vi "Configure Frequency Shift.vi"(0 "niUsrpRio session":T1 {"Daughterboard Clock Rate" format="%#.3pHz"; "FPGA Data Clock Rate" format="%#.3pHz"; "Data Clock Rate" format="%#.3pHz"; "Characterization Data"."Frequencies [Hz]" format="%#_6p"; "EEPROM Characterization Header"."Pointer to Device Data Header" format="%x"; "EEPROM Characterization Header"."Checksum" format="%x"; "Device Data Header"."Pointer to Characterization Data" format="%x"; "Device Data Header"."Checksum" format="%x"; "EEPROM Header"."Pointer to User Header" format="%x"; "EEPROM Header"."Pointer to Factory Header" format="%x"; "EEPROM Header"."Product Code" format="%x"; "EEPROM Header"."Checksum" format="%x"}, 1 "scope":string(combo)="rx/RF 0", 5 "frequency shift":dbl format="%#.3pHz", 7 "if frequency shift":dbl format="%#.3pHz", 11 "error in":errorcluster) -> (4 "niUsrpRio Session (out)":T1={"FPGA Interface"=refnum, "RIO Interface Number"=0, "Data Clock Rate"=0, "FPGA Data Clock Rate"=0, "Global Settings Register Bus"=refnum, "Radio 0 Settings Register Bus"=refnum, "Radio 1 Settings Register Bus"=refnum, "Radio Settings Bus Semaphore"=refnum, "DB Queues"=[], "Characterization Data Valid?"=FALSE, "EEPROM Header"={"Checksum"=0, "Product Code"=0, "Hardware Current Version"=0, "Hardware Oldest Compatible Version"=0, "EEPROM Map Current Version"=0, "EEPROM Map Oldest Compatible Version"=0, "User Password"="", "Pointer to Factory Header"=0, "Pointer to User Header"=0, "Recommended Interval"=0, "Number of Reserved Bytes"=9, "Number of Daughterboards"=0, "Daughterboard IDs"=[], "Daughterboard Serial Numbers"=[]}, "Device Data Header"={"Checksum"=0, "Number of Channels"=0, "Number of Gain Settings"=[], "Pointer to Characterization Data"=[], "Number of Reserved Bytes"=27, "Number of Frequencies"=[]}, "EEPROM Characterization Header"={"Checksum"=0, "Date"=timestamp(0 s since 1904-01-01), "Temperature"=0.0, "Misc. Info"="", "Pointer to Device Data Header"=0, "Number of Reserved Bytes"=28}, "Characterization Data"=[], "FPGA Current Version"=0, "FPGA Oldest Compatible Version"=0, "Fixed Logic Current Version"=0, "Fixed Logic Oldest Compatible Version"=0, "FPGA Radio Settings Bus Current Version"=0, "FPGA Radio Settings Bus Oldest Compatible Version"=0, "FPGA Board Config Current Version"=0, "FPGA Board Config Oldest Compatible Version"=0, "Daughterboard Clock Rate"=0, "daughterboard configuration session handles"=[]} {"Daughterboard Clock Rate" format="%#.3pHz"; "FPGA Data Clock Rate" format="%#.3pHz"; "Data Clock Rate" format="%#.3pHz"; "Characterization Data"."Frequencies [Hz]" format="%#_6p"; "EEPROM Characterization Header"."Pointer to Device Data Header" format="%x"; "EEPROM Characterization Header"."Checksum" format="%x"; "Device Data Header"."Pointer to Characterization Data" format="%x"; "Device Data Header"."Checksum" format="%x"; "EEPROM Header"."Pointer to User Header" format="%x"; "EEPROM Header"."Pointer to Factory Header" format="%x"; "EEPROM Header"."Product Code" format="%x"; "EEPROM Header"."Checksum" format="%x"}, 6 "coerced frequency shift":dbl format="%#.3pHz", 8 "if coerced frequency shift":dbl format="%#.3pHz", 15 "error out":errorcluster)   [LabVIEW 2018]
doc: "Configures the digital frequency shift amount.\n\n<B>Input Parameters</B>\n\n<B>niUsrpRio Session</B> is the object created by the Open VI and used as the session handle for the USRP RIO design library.\n\n<B>clock rate</B> is the frequency, in hertz, at which the DSP blocks run.\n\n<B>frequency shift</B> is the amount, in hertz, by which to shift the frequency.\n\n<B>error in</B> describes error conditions that occur before this node runs. This input provides standard 'error in' functionality.\n\n<B>Output Parameters</B>\n\n<B>error out</B> contains error information. This output provides standard 'error out' functionality."
uses:
  <instrlib>/niUsrpRio/Config/v1/Host/Public/niUsrpRio Session.ctl
  <instrlib>/_niInstr/Register Bus/v0/Host/Public/Register Bus Session.ctl
  <instrlib>/_niInstr/Register Bus/v0/Host/Private/Session Data.ctl
  <instrlib>/niUsrpRio/Config/v1/Host/Private/DB Queue Reference.ctl
  <instrlib>/niUsrpRio/Config/v1/Host/Private/Daughterboard Data.ctl
  <instrlib>/niUsrpRio/Config/v1/Host/Private/ATR state data.ctl
  <instrlib>/niUsrpRio/Config/v1/Host/Private/Antenna Configuration.ctl
  <instrlib>/niUsrpRio/Config/v1/Host/Private/CPLD Power Mode.ctl
  <instrlib>/niUsrpRio/Config/v1/Host/Public/EEPROM Header.ctl
  <instrlib>/niUsrpRio/Config/v1/Host/Public/EEPROM Device Data Header.ctl
  <instrlib>/niUsrpRio/Config/v1/Host/Public/EEPROM Characterization Header.ctl
  <instrlib>/niUsrpRio/Config/v1/Host/Public/Characterization Data.ctl
  <instrlib>/niUsrpRio/Config/v1/Host/Public/IQ Imbalance.ctl
  FPGA/SubVIs/DDC Parameters.ctl
  <instrlib>/_niInstr/DSP/v1/Shared/Public/IQ Impairments.ctl
  <vilib>/Utility/error.llb/Error Cluster From Error Code.vi
  <vilib>/rvi/errors/niLvFpgaAdjustHostInterfaceError.vi
  <vilib>/ErrorRing/Error Ring.xnode
  <vilib>/rvi/interface/nirviReadWriteControl/nirviReadWriteControl.xnode
  NiFpgaLv.dll
  <vilib>/rvi/interface/Simulation/niFpgaSimulationCallBeginRW.vi
  <instrlib>/niUsrpRio/Config/v1/Host/niUsrpRio Config v1 Host.lvlib
  <instrlib>/_niInstr/DSP/v1/Shared/niInstr DSP v1 Shared.lvlib
  <instrlib>/_niInstr/Register Bus/v0/Host/niInstr Register Bus v0 Host.lvlib
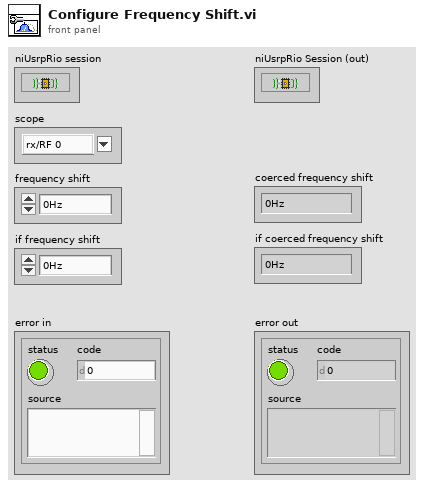
[diagram p1: front panel]
types:
  T1 = typedef "niUsrpRio Config v1 Host.lvlib/niUsrpRio Session.ctl" = cluster{"FPGA Interface":refnum<k20>, "RIO Interface Number":u32, "Data Clock Rate":u32, "FPGA Data Clock Rate":u32, "Global Settings Register Bus":T2, "Radio 0 Settings Register Bus":T2, "Radio 1 Settings Register Bus":T2, "Radio Settings Bus Semaphore":T3, "DB Queues":T4[], "Characterization Data Valid?":bool, "EEPROM Header":T5, "Device Data Header":T6, "EEPROM Characterization Header":T7, "Characterization Data":T8[], "FPGA Current Version":u32, "FPGA Oldest Compatible Version":u32, "Fixed Logic Current Version":u32, "Fixed Logic Oldest Compatible Version":u32, "FPGA Radio Settings Bus Current Version":u32, "FPGA Radio Settings Bus Oldest Compatible Version":u32, "FPGA Board Config Current Version":u32, "FPGA Board Config Oldest Compatible Version":u32, "Daughterboard Clock Rate":u32, "daughterboard configuration session handles":u64[]}
  T2 = typedef "niInstr Register Bus v0 Host.lvlib/Register Bus Session.ctl" = refnum<queue>
  T3 = typedef "Semaphore RefNum" = refnum<k1>
  T4 = typedef "niUsrpRio Config v1 Host.lvlib/DB Queue Reference.ctl" = refnum<queue>
  T5 = typedef "niUsrpRio Config v1 Host.lvlib/EEPROM Header.ctl" = cluster{"Checksum":u32, "Product Code":u16, "Hardware Current Version":u16, "Hardware Oldest Compatible Version":u16, "EEPROM Map Current Version":u16, "EEPROM Map Oldest Compatible Version":u16, "User Password":string, "Pointer to Factory Header":u32, "Pointer to User Header":u32, "Recommended Interval":u16, "Number of Reserved Bytes":i32, "Number of Daughterboards":u8, "Daughterboard IDs":u16[], "Daughterboard Serial Numbers":string[]}
  T6 = typedef "niUsrpRio Config v1 Host.lvlib/EEPROM Device Data Header.ctl" = cluster{"Checksum":u32, "Number of Channels":u8, "Number of Gain Settings":u16[], "Pointer to Characterization Data":u32[], "Number of Reserved Bytes":i32, "Number of Frequencies":u16[]}
  T7 = typedef "niUsrpRio Config v1 Host.lvlib/EEPROM Characterization Header.ctl" = cluster{"Checksum":u32, "Date":timestamp, "Temperature":sgl, "Misc. Info":string, "Pointer to Device Data Header":u32, "Number of Reserved Bytes":i32}
  T8 = typedef "niUsrpRio Config v1 Host.lvlib/Characterization Data.ctl" = cluster{"Gains[dB]":dbl[], "Frequencies [Hz]":dbl[], "IQ Imbalance Table":T9[], "Measured Gains[dB]":dbl[][]}
  T9 = typedef "niUsrpRio Config v1 Host.lvlib/IQ Imbalance.ctl" = cluster{"Gain Imbalance [linear]":dbl, "Phase Imbalance [radians]":dbl, "Offset":cdb}
  T10 = typedef "DDC Parameters.ctl" = cluster{"output sample rate":fxp<+,48,1>, "delay":fxp<+/-,16,0>, "frequency shift":fxp<+/-,48,0>, "impairments":T11, "phase":fxp<+/-,21,0>}
  T11 = typedef "niInstr DSP v1 Shared.lvlib/IQ Impairments.ctl" = cluster{"inline gain I":fxp<+/-,18,1>, "inline gain Q":fxp<+/-,18,1>, "cross gain I":fxp<+/-,18,1>, "cross gain Q":fxp<+/-,18,1>, "pre-gain offset I":fxp<+/-,18,1>, "pre-gain offset Q":fxp<+/-,18,1>, "post-gain offset I":fxp<+/-,18,1>, "post-gain offset Q":fxp<+/-,18,1>}
  T12 = typedef "niUsrpRio Config v1 Host.lvlib/Device Subfunction.ctl" = enum16{"rx", "tx", "all"}
  T13 = typedef "niUsrpRio Config v1 Host.lvlib/RF Channel 2.ctl" = enum16{"0", "1", "2", "3", "All"}
  T14 = typedef "niUsrpRio Config v1 Host.lvlib/DB Types.ctl" = enum16{"sbx", "cbx", "wbx", "unknown", "ubx", "twinrx"}
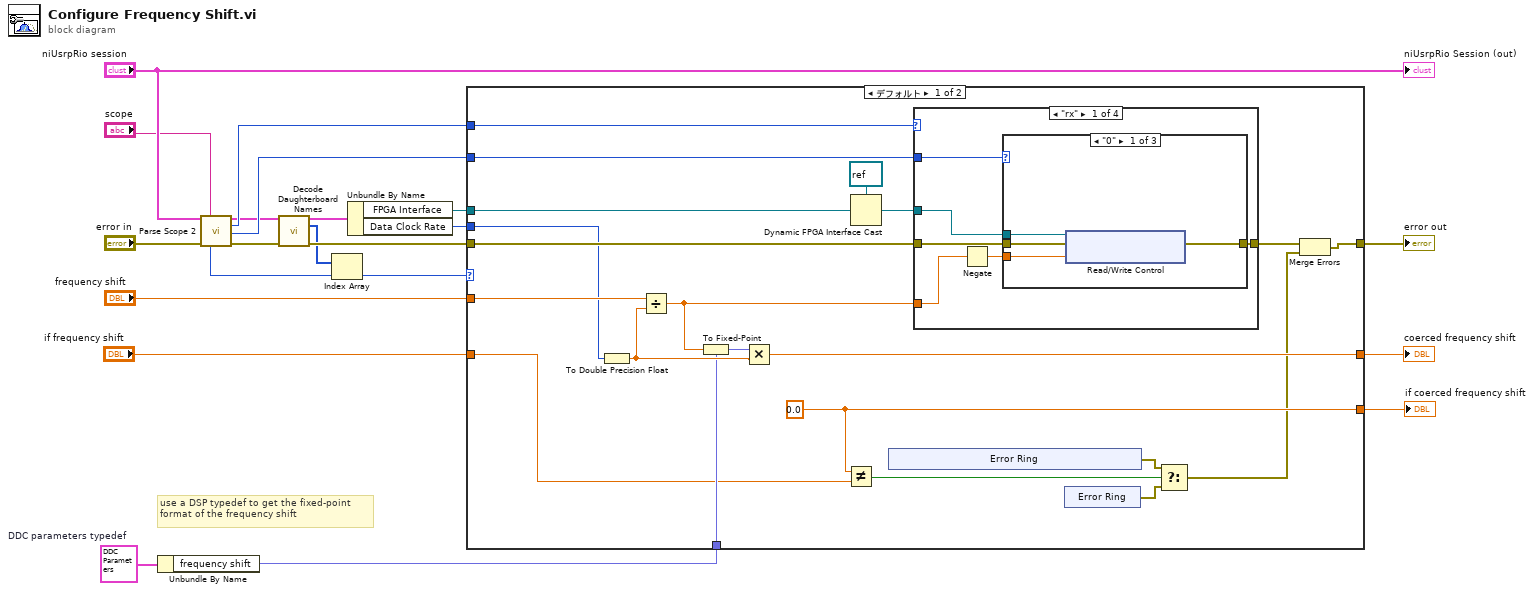
[diagram p0: block diagram]
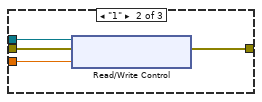
[diagram p2: hidden frame]
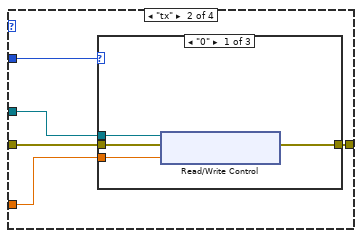
[diagram p4: hidden frame]
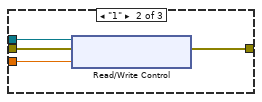
[diagram p5: hidden frame]
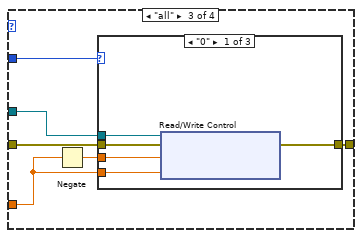
[diagram p7: hidden frame]
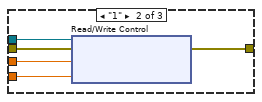
[diagram p8: hidden frame]
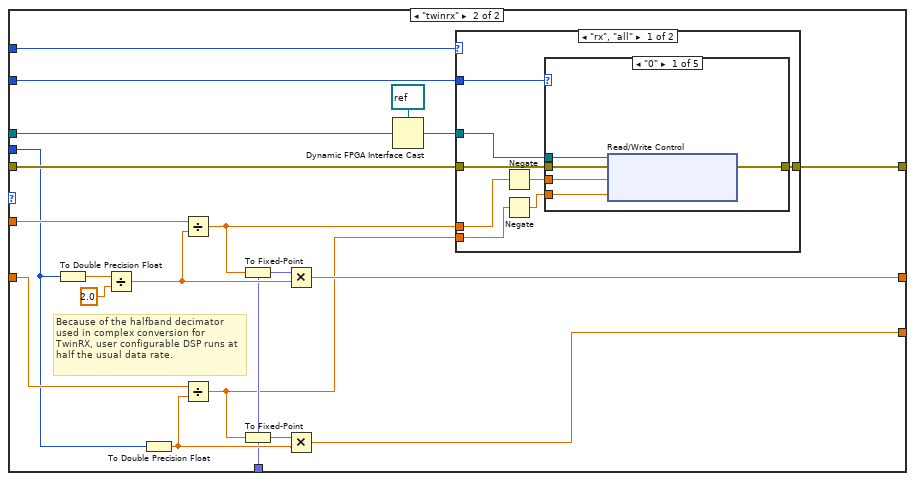
[diagram p11: hidden frame]
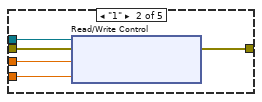
[diagram p12: hidden frame]
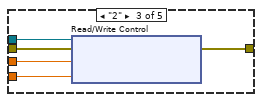
[diagram p13: hidden frame]
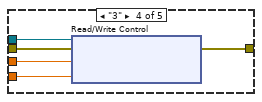
[diagram p14: hidden frame]
diagram:
  w19 = T10 {"output sample rate"=1.0, "delay"=0.0, "frequency shift"=0.0, "impairments"={"inline gain I"=0.9999923706054688, "inline gain Q"=0.9999923706054688, "cross gain I"=0.0, "cross gain Q"=0.0, "pre-gain offset I"=0.0, "pre-gain offset Q"=0.0, "post-gain offset I"=0.0, "post-gain offset Q"=0.0}, "phase"=0.0}  # DDC parameters typedef
  # "use a DSP typedef to get the fixed-point format of the frequency shift"
  n1 = Unbundle By Name(w19) -> ("frequency shift"=w6:fxp<+/-,48,0>)
  n2 = call <instrlib>:"Parse Scope 2.vi"("niUsrpRio Session"="niUsrpRio session", "scope"="scope", "error in"="error in") -> ("niUsrpRio Session (out)"=w12:T1, "Device Subfunction"=w16:T12, "Device Subfunction Channel"=w21:T13, "daughterboard index"=w9:u32, "error out"=w17:errorcluster)  [unwired: 4 in, 4 out]
  n3 = call <instrlib>:"Decode Daughterboard Names.vi"("niUsrpRio Session"=w12, "error in"=w17) -> ("niUsrpRio Session (out)"=w11:T1, "daughterboard names"=w10:T14[], "error out"=w13:errorcluster)  [unwired: 10 in, 1 out]
  n4 = Index Array(array=w10, index=w9) -> (element=w8:T14)
  n5 = Unbundle By Name(w11) -> ("FPGA Interface"=w7:refnum<k20>, "Data Clock Rate"=w2:u32)
  n6 = case shown="デフォルト" w8 {
    tunnel: w21 -> [w42 w116]
    tunnel: [w24 w115] -> w20
    tunnel: w7 -> [w39 w111]
    tunnel: w16 -> [w41 w114]
    tunnel: w13 -> [w40 w113]
    tunnel: w6 -> [w31 w103]
    tunnel: "if frequency shift" -> [w28 w104]
    tunnel: "frequency shift" -> [w34 w102]
    tunnel: [w32 w101] -> w3
    tunnel: w2 -> [w33 w98]
    tunnel: [w29 w96] -> w1
    frame Default {
      w29 = 0.0
      n7 = To Double Precision Float(number=w33) -> (double precision float=w36:dbl)
      n8 = Divide(x=w34, y=w36) -> (x/y=w30:dbl)
      n9 = To Fixed-Point(fixed-point type=w31, number=w30) -> (fixed-point=w35:fxp<+/-,48,0>)
      n10 = Multiply(x=w35, y=w36) -> (x*y=w32:dbl)
      n11 = Not Equal?(x=w29, y=w28) -> (x != y?=w27:bool)
      n12 = Dynamic FPGA Interface Cast(Session In=refnum<k20> refnum ("FPGA VI Reference Out"), Type=w39) -> (Session Out=w38:refnum<k20>)
      n13 = xnode "Error Ring"() -> ("エラー出力"=w26:errorcluster)
      n14 = case shown="\"rx\"" w41 {
        tunnel: w38 -> [w50 w68 w79 _]
        tunnel: [w54 w67 w83 w95] -> w23
        tunnel: w40 -> [w53 w66 w82 w95]
        tunnel: w42 -> [w51 w65 w80 _]
        tunnel: w30 -> [w49 w64 w78 _]
        frame "rx" {
          n15 = Negate(x=w49) -> (-x=w52:dbl)
          n16 = case shown="\"0\"" w51 {
            tunnel: w50 -> [w58 w62 _]
            tunnel: [w57 w61 w63] -> w54
            tunnel: w53 -> [w56 w60 w63]
            tunnel: w52 -> [w55 w59 _]
            frame "0" {
              n17 = xnode "Read/Write Control"("FPGA VIリファレンス入力"=w58, "エラー入力"=w56, "rx 0.frequency shift"=w55) -> ("エラー出力"=w57:errorcluster)  [unwired: 1 out]
            }
            frame "1" {
              n18 = xnode "Read/Write Control"("FPGA VIリファレンス入力"=w62, "エラー入力"=w60, "rx 1.frequency shift"=w59) -> ("エラー出力"=w61:errorcluster)  [unwired: 1 out]
            }
            frame Default {
            }
          }
        }
        frame "tx" {
          n19 = case shown="\"0\"" w65 {
            tunnel: w68 -> [w72 w76 _]
            tunnel: [w71 w75 w77] -> w67
            tunnel: w66 -> [w70 w74 w77]
            tunnel: w64 -> [w69 w73 _]
            frame "0" {
              n20 = xnode "Read/Write Control"("FPGA VIリファレンス入力"=w72, "エラー入力"=w70, "tx 0.frequency shift"=w69) -> ("エラー出力"=w71:errorcluster)  [unwired: 1 out]
            }
            frame "1" {
              n21 = xnode "Read/Write Control"("FPGA VIリファレンス入力"=w76, "エラー入力"=w74, "tx 1.frequency shift"=w73) -> ("エラー出力"=w75:errorcluster)  [unwired: 1 out]
            }
            frame Default {
            }
          }
        }
        frame "all" {
          n22 = Negate(x=w78) -> (-x=w81:dbl)
          n23 = case shown="\"0\"" w80 {
            tunnel: w79 -> [w88 w93 _]
            tunnel: [w87 w92 w94] -> w83
            tunnel: w82 -> [w86 w91 w94]
            tunnel: w81 -> [w85 w90 _]
            tunnel: w78 -> [w84 w89 _]
            frame "0" {
              n24 = xnode "Read/Write Control"("FPGA VIリファレンス入力"=w88, "エラー入力"=w86, "rx 0.frequency shift"=w85, "tx 0.frequency shift"=w84) -> ("エラー出力"=w87:errorcluster)  [unwired: 1 out]
            }
            frame "1" {
              n25 = xnode "Read/Write Control"("FPGA VIリファレンス入力"=w93, "エラー入力"=w91, "rx 1.frequency shift"=w90, "tx 1.frequency shift"=w89) -> ("エラー出力"=w92:errorcluster)  [unwired: 1 out]
            }
            frame Default {
            }
          }
        }
        frame Default {
        }
      }
      n26 = xnode "Error Ring"() -> ("エラー出力"=w25:errorcluster)
      n27 = Select(t=w26, s=w27, f=w25) -> (s? t:f=w22:errorcluster)
      n28 = Merge Errors(w23, w22) -> (w24:errorcluster)
    }
    frame "twinrx" {
      # "Because of the halfband decimator used in complex conversion for TwinRX, user configurable DSP runs at half the usual data rate."
      n29 = To Double Precision Float(number=w98) -> (double precision float=w99:dbl)
      n30 = Divide(x=w99, y=2.0) -> (x/y=w107:dbl)
      n31 = To Double Precision Float(number=w98) -> (double precision float=w108:dbl)
      n32 = Divide(x=w102, y=w107) -> (x/y=w100:dbl)
      n33 = Divide(x=w104, y=w108) -> (x/y=w97:dbl)
      n34 = To Fixed-Point(fixed-point type=w103, number=w100) -> (fixed-point=w106:fxp<+/-,48,0>)
      n35 = To Fixed-Point(fixed-point type=w103, number=w97) -> (fixed-point=w109:fxp<+/-,48,0>)
      n36 = Multiply(x=w106, y=w107) -> (x*y=w101:dbl)
      n37 = Multiply(x=w109, y=w108) -> (x*y=w96:dbl)
      n38 = Dynamic FPGA Interface Cast(Session In=refnum<k20> refnum ("FPGA VI Reference Out"), Type=w111) -> (Session Out=w112:refnum<k20>)
      n39 = case shown="\"rx\", \"all\"" w114 {
        tunnel: w100 -> [w120 _]
        tunnel: w112 -> [w121 _]
        tunnel: [w124 w146] -> w115
        tunnel: w113 -> [w123 w146]
        tunnel: w116 -> [w122 _]
        tunnel: w97 -> [w117 _]
        frame "rx", "all" {
          n40 = Negate(x=w120) -> (-x=w119:dbl)
          n41 = Negate(x=w117) -> (-x=w118:dbl)
          n42 = case shown="\"0\"" w122 {
            tunnel: w121 -> [w129 w134 w139 w144 _]
            tunnel: [w128 w133 w138 w143 w145] -> w124
            tunnel: w123 -> [w127 w132 w137 w142 w145]
            tunnel: w119 -> [w126 w131 w136 w141 _]
            tunnel: w118 -> [w125 w130 w135 w140 _]
            frame "0" {
              n43 = xnode "Read/Write Control"("FPGA VIリファレンス入力"=w129, "エラー入力"=w127, "rx 0.frequency shift"=w126, "rx 0.if frequency shift"=w125) -> ("エラー出力"=w128:errorcluster)  [unwired: 1 out]
            }
            frame "1" {
              n44 = xnode "Read/Write Control"("FPGA VIリファレンス入力"=w134, "エラー入力"=w132, "rx 1.frequency shift"=w131, "rx 1.if frequency shift"=w130) -> ("エラー出力"=w133:errorcluster)  [unwired: 1 out]
            }
            frame "2" {
              n45 = xnode "Read/Write Control"("FPGA VIリファレンス入力"=w139, "エラー入力"=w137, "rx 2.frequency shift"=w136, "rx 2.if frequency shift"=w135) -> ("エラー出力"=w138:errorcluster)  [unwired: 1 out]
            }
            frame "3" {
              n46 = xnode "Read/Write Control"("FPGA VIリファレンス入力"=w144, "エラー入力"=w142, "rx 3.frequency shift"=w141, "rx 3.if frequency shift"=w140) -> ("エラー出力"=w143:errorcluster)  [unwired: 1 out]
            }
            frame Default {
            }
          }
        }
        frame Default {
        }
      }
    }
  }
  "error out" <- w20
  "coerced frequency shift" <- w3
  "if coerced frequency shift" <- w1
  "niUsrpRio Session (out)" <- "niUsrpRio session"
